vi "Create.vi"(0 "MLA":refnum<class "MLA.lvclass">, 1 "Application Name":string, 2 "Application Version":string, 3 "Revision History":string, 5 "error in (no error)":errorcluster, 8 "VI Reference":refnum<vi>) -> (14 "MLA":refnum<class "MLA.lvclass">, 19 "error out":errorcluster)   [LabVIEW 2017, in "MLA.lvclass"]
uses:
  MLA.lvclass
  controls/MLA Loops.ctl
  MLA Stop Mode.ctl
  S5Tools/ErrorLog/ErrorLog.lvclass
panel:
  in  "MLA Loops Typedef":T1
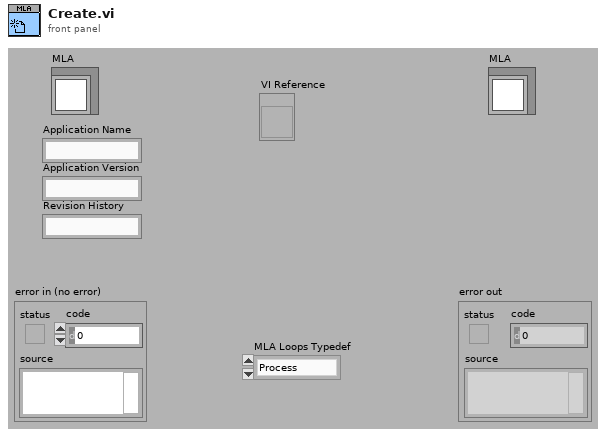
[diagram p1: front panel]
types:
  T1 = typedef "MLA Loops.ctl" = enum16{"Process", "SendToRT", "ReceiveFromRT", "FileTransfer", "Script"}
  T2 = typedef "MLA Stop Mode.ctl" = enum16{"Read", "Set", "Reset"}
  T3 = typedef "MLA.lvclass/ObjectAttributes.ctl" = cluster{"App Name":string, "App Version":string, "Revision History":string, "Log File Path":path, "Config INI File":path, "Config Path":path, "Log Archive Path":path, "Msg Q's":refnum<queue>[], "VI":refnum<vi>, "ErrLog":refnum<class "ErrorLog.lvclass">}
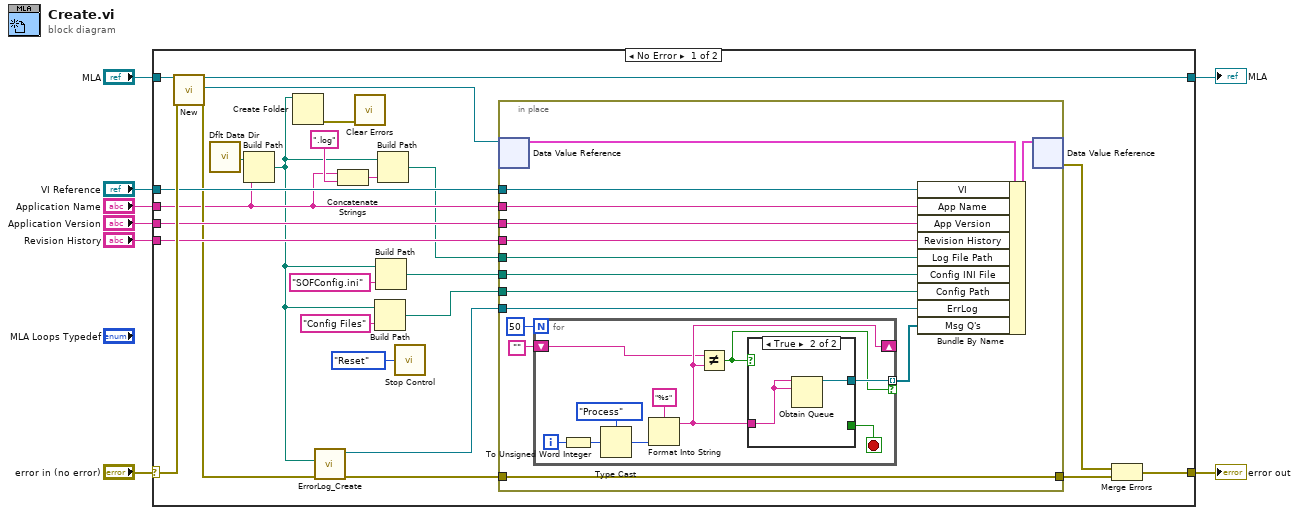
[diagram p0: block diagram]
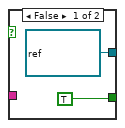
[diagram p2: hidden frame]
diagram:
  n1 = case shown="No Error" "error in (no error)" {
    selector: "error in (no error)" -> [w32 w63]
    tunnel: [w29 w63] -> w7
    tunnel: "MLA" -> [w33 w62]
    tunnel: [w31 w62] -> w5
    tunnel: "VI Reference" -> [w23 _]
    tunnel: "Application Name" -> [w14 _]
    tunnel: "Application Version" -> [w18 _]
    tunnel: "Revision History" -> [w17 _]
    frame No Error {
      n2 = call "New.vi"("MLA"=w33, "error in (no error)"=w32) -> ("MLA"=w31:refnum<class "MLA.lvclass">, "DVRRefOut"=w20:refnum<data-value>, "error out"=w16:errorcluster)  [unwired: 14 in, 1 out]
      n3 = call <vilib>:"Dflt Data Dir.vi"() -> ("App:Default Data Directory"=w21:path)
      n4 = Build Path(base path=w21, name or relative path=w14) -> (appended path=w10:path)
      n5 = Create Folder(path (use dialog)=w10) -> (error out=w9:errorcluster)  [unwired: 2 in, 2 out]
      n6 = call "ErrorLog_Create.vi"("error in (no error)"=w16, "ErrorLog Folder (c:\\)"=w10) -> ("error out"=w15:errorcluster, "reference out"=w13:refnum<class "ErrorLog.lvclass">)  [unwired: 8 in]
      n7 = Concatenate Strings(w14, ".log" ("name or relative path")) -> (w22:string)
      n8 = call <vilib>:"Clear Errors.vi"("error in (no error)"=w9) -> ()  [unwired: 5 in, 2 out]
      n9 = Build Path(base path=w10, name or relative path="Config Files") -> (appended path=w24:path)
      n10 = Build Path(base path=w10, name or relative path="SOFConfig.ini") -> (appended path=w26:path)
      n11 = Build Path(base path=w10, name or relative path=w22) -> (appended path=w12:path)
      n12 = call "Stop Control.vi"("Mode (Read)"=MLA_Stop_Mode."Reset" ("Mode")) -> ()  [unwired: 1 out]
      n13 = in-place {
        in-place-border: w15 -> [w43]
        in-place-border: [w43] -> w28
        in-place-border: w26 -> [w45]
        in-place-border: w24 -> [w44]
        in-place-border: w23 -> [w42]
        in-place-border: w14 -> [w41]
        in-place-border: w18 -> [w40]
        in-place-border: w17 -> [w39]
        in-place-border: w13 -> [w37]
        in-place-border: w12 -> [w36]
        n14 = in-place-dvr #1(w20) -> (w46:T3)  [unwired: 1 out]
        n15 = for {
          N: 50 -> [_]
          tunnel: [w57] -> w38 mode=indexing if=w50
          shift-right: [w49] -> _
          shift-left: "" -> [w48]
          i -> [w52]
          stop <- w51 stop-if-true
          n16 = To Unsigned Word Integer(number=w52) -> (unsigned 16bit integer=w53:u16)
          n17 = Type Cast(type=MLA_Loops."Process" ("MLA Loops Typedef"), x=w53) -> (*(type *) &x=w56:T1)
          n18 = Format Into String(format string="%s", w56) -> (resulting string=w49:string)  [unwired: 2 in, 1 out]
          n19 = Not Equal?(x=w48, y=w49) -> (x != y?=w50:bool)
          n20 = case shown="True" w50 {
            tunnel: [refnum<queue> refnum ("queue out") w61] -> w57
            tunnel: [TRUE _] -> w51
            tunnel: w49 -> [_ w60]
            frame False {
            }
            frame True {
              n21 = Obtain Queue(name (unnamed)=w60, element data type=w60) -> (queue out=w61:refnum<queue>)  [unwired: 3 in, 2 out]
            }
          }
        }
        n22 = Bundle By Name(cluster=w46, "VI"=w42, "App Name"=w41, "App Version"=w40, "Revision History"=w39, "Log File Path"=w36, "Config INI File"=w45, "Config Path"=w44, "ErrLog"=w37, "Msg Q's"=w38) -> (w47:T3)
        n23 = in-place-dvr #1(w47) -> (w30:errorcluster)  [unwired: 1 out]
      }
      n24 = Merge Errors(w30, w28) -> (w29:errorcluster)
    }
    frame Error {
    }
  }
  "error out" <- w7
  "MLA" <- w5
